vi "Event Start.vi"(7 "Event Name":string, 8 "error in":errorcluster) -> (0 "error out":errorcluster)   [LabVIEW 2027, in "VS Tracing API.lvlib"]
doc: "Records the start of a user-space event on the current timed structure thread. The event remains active until the corresponding <i>Event Stop</i> is called.\nUse this VI inside Timed Loops, Timed Sequences, or other timed execution contexts where timing information should be associated with the current execution thread.\n\n<b>Parameters</b>\n• <b>Event Name</b>: Name of the event to be displayed in the trace.\n\n<b>Notes</b>\n• Must be paired with <i>Event Stop</i>.\n• The event appears on the track corresponding to the timed structure in which it is executed."
uses:
  VS Tracing API.lvlib
  libvs_perfetto.dll
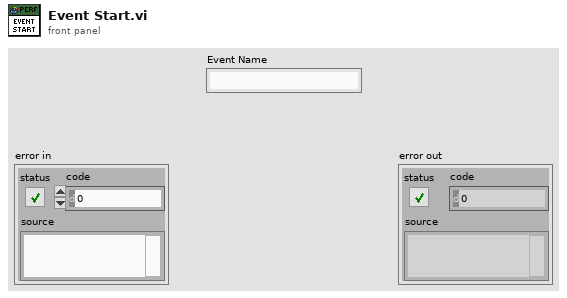
[diagram p1: front panel]
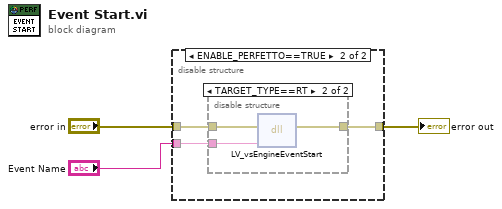
[diagram p0: block diagram]
diagram:
  n1 = disable-structure shown="ENABLE_PERFETTO==TRUE" {
    disable-tunnel: "Event Name" -> [_ w5]
    disable-tunnel: "error in" -> [w4 w6]
    disable-tunnel: [w4 w7] -> w2
    frame condition #0 (active) {
    }
    frame condition #1 {
      n2 = disable-structure shown="TARGET_TYPE==RT" {
        disable-tunnel: [w8 w11] -> w7
        disable-tunnel: w6 -> [w8 w10]
        disable-tunnel: w5 -> [_ w9]
        frame condition #0 (active) {
        }
        frame condition #1 {
          n3 = dll-call lib="libvs_perfetto.*" fn="LV_vsEngineEventStart"(error in=w10, "eventName"=w9) -> (error out=w11:errorcluster)  [unwired: 4 in, 1 out]
        }
      }
    }
  }
  "error out" <- w2
